vi "Initialize.vi"(8 "error in (no error)":errorcluster caption="错误输入（无错误）", 11 "Item输入":refnum<class "Item.lvclass">) -> (0 "error out":errorcluster caption="错误输出", 3 "Item输出":refnum<class "Item.lvclass">)   [LabVIEW 2013, in "Hierarchy Framework.lvlib" / "Item.lvclass"]
uses:
  Item.lvclass
  Generic/Generic.lvclass
  Item.lvclass/Item.ctl
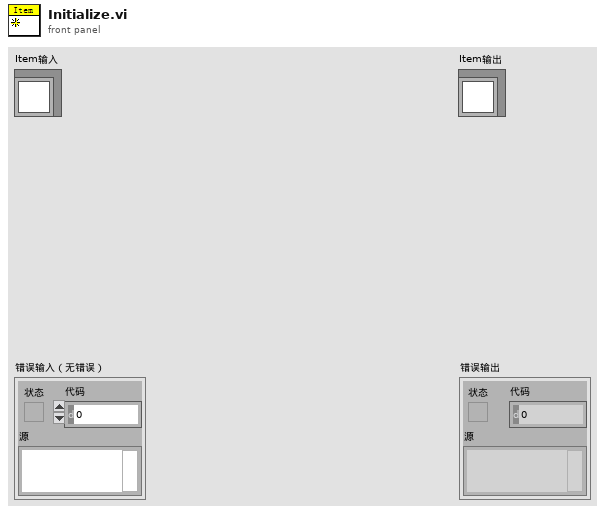
[diagram p1: front panel]
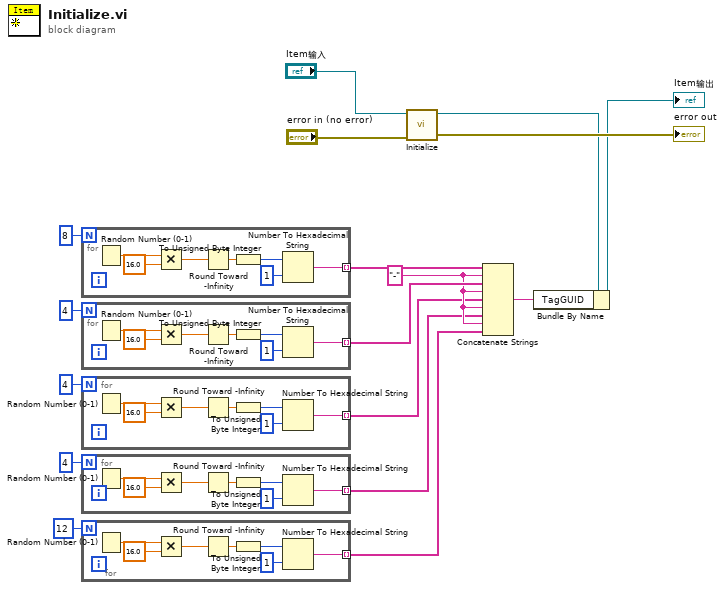
[diagram p0: block diagram]
diagram:
  w7 = "-" ("string")
  n1 = for {
    N: 8 -> [_]
    tunnel: [w18] -> w9 mode=indexing
    n2 = Random Number (0-1)() -> (number: 0 to 1=w24:dbl)
    n3 = Multiply(x=w24, y=16.0) -> (x*y=w22:dbl)
    n4 = Round Toward -Infinity(1:w22) -> (0:w21:dbl)
    n5 = To Unsigned Byte Integer(number=w21) -> (unsigned 8bit integer=w20:u8)
    n6 = Number To Hexadecimal String(1:i16 1 ("width (-)"), 2:w20) -> (0:w18:string)
  }
  n7 = for {
    N: 4 -> [_]
    tunnel: [w25] -> w8 mode=indexing
    n8 = Random Number (0-1)() -> (number: 0 to 1=w31:dbl)
    n9 = Multiply(x=w31, y=16.0) -> (x*y=w29:dbl)
    n10 = Round Toward -Infinity(1:w29) -> (0:w28:dbl)
    n11 = To Unsigned Byte Integer(number=w28) -> (unsigned 8bit integer=w27:u8)
    n12 = Number To Hexadecimal String(1:i16 1 ("width (-)"), 2:w27) -> (0:w25:string)
  }
  n13 = for {
    N: 4 -> [_]
    tunnel: [w32] -> w6 mode=indexing
    n14 = Random Number (0-1)() -> (number: 0 to 1=w38:dbl)
    n15 = Multiply(x=w38, y=16.0) -> (x*y=w36:dbl)
    n16 = Round Toward -Infinity(1:w36) -> (0:w35:dbl)
    n17 = To Unsigned Byte Integer(number=w35) -> (unsigned 8bit integer=w34:u8)
    n18 = Number To Hexadecimal String(1:i16 1 ("width (-)"), 2:w34) -> (0:w32:string)
  }
  n19 = for {
    N: 4 -> [_]
    tunnel: [w39] -> w5 mode=indexing
    n20 = Random Number (0-1)() -> (number: 0 to 1=w45:dbl)
    n21 = Multiply(x=w45, y=16.0) -> (x*y=w43:dbl)
    n22 = Round Toward -Infinity(1:w43) -> (0:w42:dbl)
    n23 = To Unsigned Byte Integer(number=w42) -> (unsigned 8bit integer=w41:u8)
    n24 = Number To Hexadecimal String(1:i16 1 ("width (-)"), 2:w41) -> (0:w39:string)
  }
  n25 = for {
    N: 12 -> [_]
    tunnel: [w46] -> w4 mode=indexing
    n26 = Random Number (0-1)() -> (number: 0 to 1=w52:dbl)
    n27 = Multiply(x=w52, y=16.0) -> (x*y=w50:dbl)
    n28 = Round Toward -Infinity(1:w50) -> (0:w49:dbl)
    n29 = To Unsigned Byte Integer(number=w49) -> (unsigned 8bit integer=w48:u8)
    n30 = Number To Hexadecimal String(1:i16 1 ("width (-)"), 2:w48) -> (0:w46:string)
  }
  n31 = call-parent "Initialize.vi"("error in (no error)"="error in (no error)", "Generic输入"="Item输入") -> ("error out"=→"error out":errorcluster, "Generic输出"=w3:refnum<class "Item.lvclass">)  [unwired: 8 in]
  n32 = Concatenate Strings(w9, w7, w8, w7, w6, w7, w5, w7, w4) -> (w1:string)
  n33 = Bundle By Name(cluster=w3, "TagGUID"=w1) -> (→"Item输出":refnum<class "Item.lvclass">)
